vi "From Variant.vi"(8 "Error In":errorcluster, 10 "Variant":variant, 11 "Tree Data In":refnum<class "Tree Data.lvclass">) -> (0 "Error Out":errorcluster, 3 "Tree Data Out":refnum<class "Tree Data.lvclass">)   [LabVIEW 2017, in "Tree API.lvlib" / "Tree Data.lvclass"]
doc: "Dynamic dispatch interface for conversion of variant LV data to Tree Data classes."
uses:
  Tree Data.lvclass
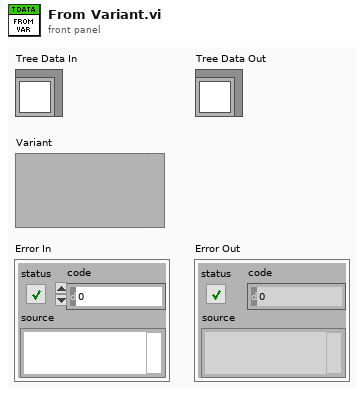
[diagram p1: front panel]
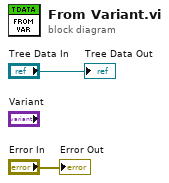
[diagram p0: block diagram]
diagram:
  "Error Out" <- "Error In"
  "Tree Data Out" <- "Tree Data In"
